vi "ke37xx DAC-Totalizer Calibration.vi"() -> ()   [LabVIEW 2009, in "Keithley 3700 Series.lvlib"]
doc: "This VI provides a way to calibrate the 3750 Digital I/O Card's DAC and totalizer channels. Ensure all inputs to the channels being calibrated are disconnected."
uses:
  <instrlib>/Keithley 3706/Keithley 3700 Series.lvlib
panel:
  out "Calibration Failed":bool=TRUE
  out "Calibration Completed":bool
  out "error out":errorcluster
  in  "Calibration Password":string
  in  "Channel Type":enum32{"Radio Selection 1", "Radio Selection 2"}(radio)
  in  "Channel to Calibrate":string
  in  "VISA Resource Name":refnum<visa-resource-name>
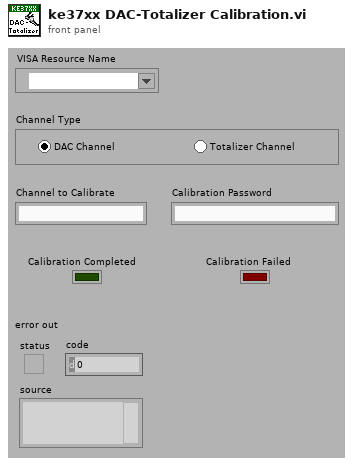
[diagram p1: front panel]
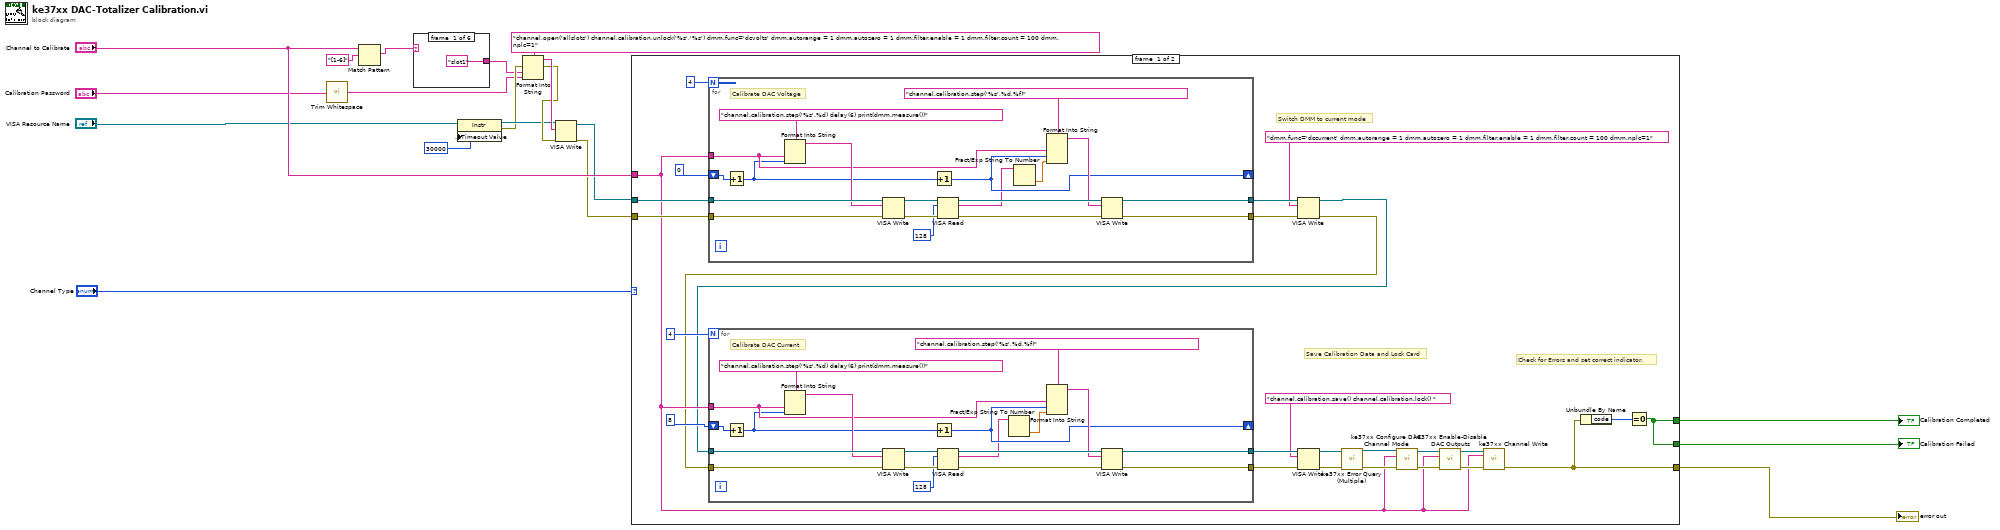
[diagram p0: block diagram]
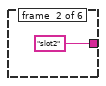
[diagram p2: hidden frame]
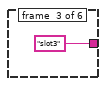
[diagram p3: hidden frame]
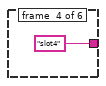
[diagram p4: hidden frame]
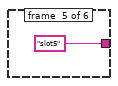
[diagram p5: hidden frame]
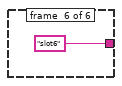
[diagram p6: hidden frame]
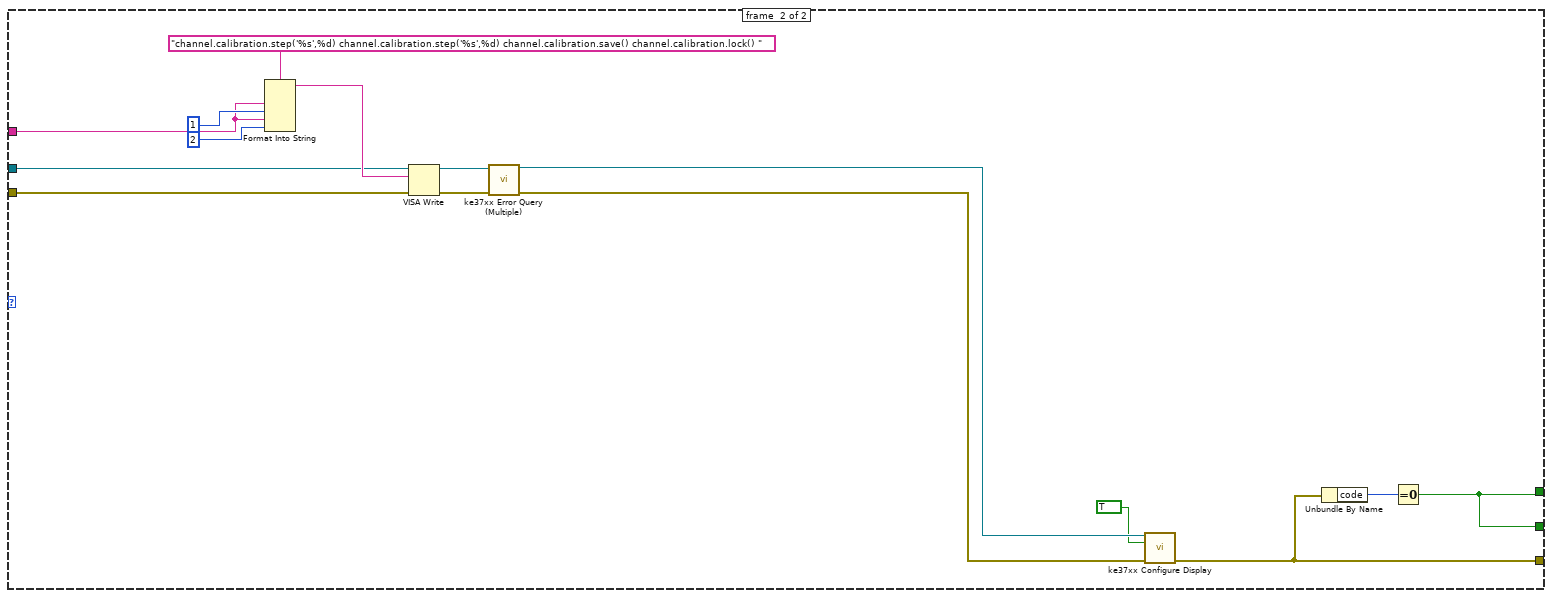
[diagram p7: hidden frame]
diagram:
  n1 = call <vilib>:"Trim Whitespace.vi"("string"="Calibration Password") -> ("trimmed string"=w1:string)  [unwired: 1 in]
  n2 = Match Pattern(string="Channel to Calibrate", regular expression="[1-6]") -> (match substring=w6:string)  [unwired: 4 out]
  n3 = case shown="\"4\"" w6 {
    tunnel: ["slot1" "slot2" "slot3" "slot4" "slot5" "slot6"] -> w5
    frame #0 {
    }
    frame #1 {
    }
    frame #2 {
    }
    frame #3 {
    }
    frame #4 {
    }
    frame #5 {
    }
  }
  n4 = property class="Instr"(reference="VISA Resource Name", "General Settings:Timeout Value"=u32 30000) -> (reference out=w9:refnum<visa-resource-name>, error out=w8:errorcluster)  [unwired: 1 in]
  n5 = Format Into String(format string="channel.open('allslots') channel.calibration.unlock('%s','%s') dmm.func='dcvolts' dmm.autorange = 1 dmm.autozero = 1 dmm.filter.enable = 1 dmm.filter.count = 100 dmm.nplc=1", error in=w8, w5, w1) -> (resulting string=w13:string, error out=w10:errorcluster)  [unwired: 1 in]
  n6 = VISA Write(VISA resource name=w9, write buffer=w13, error in (no error)=w10) -> (VISA resource name out=w4:refnum<visa-resource-name>, error out=w3:errorcluster)  [unwired: 1 out]
  n7 = case shown="\"Radio Selection 1\", Default" "Channel Type" {
    tunnel: w3 -> [w50 w101]
    tunnel: w4 -> [w49 w102]
    tunnel: "Channel to Calibrate" -> [w32 w96]
    tunnel: [w26 w93] -> w14
    tunnel: [w27 w94] -> w16
    tunnel: [w27 w94] -> w15
    frame #0 {
      # "Check for Errors and set correct indicator."
      # "Switch DMM to current mode"
      # "Save Calibration Data and Lock Card"
      n8 = for {
        N: 4 -> [_]
        tunnel: [w71] -> w46
        tunnel: w50 -> [w89]
        tunnel: w49 -> [w88]
        tunnel: w32 -> [w78]
        shift-right: [w77] -> _
        shift-left: 0 -> [w75]
        tunnel: [w72] -> w47
        # "Calibrate DAC Voltage"
        n9 = Increment(x=w75) -> (x+1=w76:i32)
        n10 = Format Into String(format string="channel.calibration.step('%s',%d) delay(6) print(dmm.measure())", w78, w76) -> (resulting string=w86:string)  [unwired: 2 in, 1 out]
        n11 = VISA Write(VISA resource name=w88, write buffer=w86, error in (no error)=w89) -> (VISA resource name out=w85:refnum<visa-resource-name>, error out=w84:errorcluster)  [unwired: 1 out]
        n12 = Increment(x=w76) -> (x+1=w77:i32)
        n13 = VISA Read(VISA resource name=w85, byte count=128, error in (no error)=w84) -> (VISA resource name out=w82:refnum<visa-resource-name>, read buffer=w74:string, error out=w81:errorcluster)  [unwired: 1 out]
        n14 = Fract/Exp String To Number(string=w74) -> (number=w73:dbl)  [unwired: 4 out]
        n15 = Format Into String(format string="channel.calibration.step('%s',%d,%f)", w78, w77, w73) -> (resulting string=w79:string)  [unwired: 2 in, 1 out]
        n16 = VISA Write(VISA resource name=w82, write buffer=w79, error in (no error)=w81) -> (VISA resource name out=w72:refnum<visa-resource-name>, error out=w71:errorcluster)  [unwired: 1 out]
      }
      n17 = VISA Write(VISA resource name=w47, write buffer="dmm.func='dccurrent' dmm.autorange = 1 dmm.autozero = 1 dmm.filter.enable = 1 dmm.filter.count = 100 dmm.nplc=1", error in (no error)=w46) -> (VISA resource name out=w29:refnum<visa-resource-name>, error out=w28:errorcluster)  [unwired: 1 out]
      n18 = for {
        N: 4 -> [_]
        tunnel: [w53] -> w31
        tunnel: w28 -> [w70]
        tunnel: w29 -> [w69]
        tunnel: w32 -> [w59]
        shift-right: [w58] -> _
        shift-left: 8 -> [w56]
        tunnel: [w54] -> w40
        # "Calibrate DAC Current"
        n19 = Increment(x=w56) -> (x+1=w57:i32)
        n20 = Format Into String(format string="channel.calibration.step('%s',%d) delay(6) print(dmm.measure())", w59, w57) -> (resulting string=w67:string)  [unwired: 2 in, 1 out]
        n21 = VISA Write(VISA resource name=w69, write buffer=w67, error in (no error)=w70) -> (VISA resource name out=w66:refnum<visa-resource-name>, error out=w65:errorcluster)  [unwired: 1 out]
        n22 = Increment(x=w57) -> (x+1=w58:i32)
        n23 = VISA Read(VISA resource name=w66, byte count=128, error in (no error)=w65) -> (VISA resource name out=w63:refnum<visa-resource-name>, read buffer=w55:string, error out=w62:errorcluster)  [unwired: 1 out]
        n24 = Fract/Exp String To Number(string=w55) -> (number=w52:dbl)  [unwired: 4 out]
        n25 = Format Into String(format string="channel.calibration.step('%s',%d,%f)", w59, w58, w52) -> (resulting string=w60:string)  [unwired: 2 in, 1 out]
        n26 = VISA Write(VISA resource name=w63, write buffer=w60, error in (no error)=w62) -> (VISA resource name out=w54:refnum<visa-resource-name>, error out=w53:errorcluster)  [unwired: 1 out]
      }
      n27 = VISA Write(VISA resource name=w40, write buffer="channel.calibration.save() channel.calibration.lock() ", error in (no error)=w31) -> (VISA resource name out=w41:refnum<visa-resource-name>, error out=w42:errorcluster)  [unwired: 1 out]
      n28 = call <instrlib>:"ke37xx Error Query (Multiple).vi"("VISA resource name"=w41, "error in (no error)"=w42) -> ("VISA resource name out"=w38:refnum<visa-resource-name>, "error out"=w37:errorcluster)  [unwired: 12 out]
      n29 = call <instrlib>:"ke37xx Configure DAC Channel Mode.vi"("error in (no error)"=w37, "DAC Channels"=w32, "VISA Resource Name"=w38) -> ("error out"=w35:errorcluster, "VISA Resource Name Out"=w36:refnum<visa-resource-name>)  [unwired: 1 in, 6 out]
      n30 = call <instrlib>:"ke37xx Enable-Disable DAC Outputs.vi"("error in (no error)"=w35, "Channel"=w32, "VISA Resource Name"=w36) -> ("error out"=w33:errorcluster, "VISA Resource Name Out"=w34:refnum<visa-resource-name>)  [unwired: 1 in, 6 out]
      n31 = call <instrlib>:"ke37xx Channel Write.vi"("VISA Resource Name"=w34, "Channel"=w32, "error in (no error)"=w33) -> ("error out"=w26:errorcluster)  [unwired: 2 in, 10 out]
      n32 = Unbundle By Name(w26) -> ("code"=w30:i32)
      n33 = Equal To 0?(x=w30) -> (x = 0?=w27:bool)
    }
    frame #1 {
      n34 = Format Into String(format string="channel.calibration.step('%s',%d) channel.calibration.step('%s',%d) channel.calibration.save() channel.calibration.lock() ", w96, 1, w96, 2) -> (resulting string=w103:string)  [unwired: 2 in, 1 out]
      n35 = VISA Write(VISA resource name=w102, write buffer=w103, error in (no error)=w101) -> (VISA resource name out=w99:refnum<visa-resource-name>, error out=w98:errorcluster)  [unwired: 1 out]
      n36 = call <instrlib>:"ke37xx Error Query (Multiple).vi"("VISA resource name"=w99, "error in (no error)"=w98) -> ("VISA resource name out"=w91:refnum<visa-resource-name>, "error out"=w92:errorcluster)  [unwired: 12 out]
      n37 = call <instrlib>:"ke37xx Configure Display.vi"("VISA Resource Name"=w91, "Clear Display (False)"=TRUE, "error in (no error)"=w92) -> ("error out"=w93:errorcluster)  [unwired: 11 in, 1 out]
      n38 = Unbundle By Name(w93) -> ("code"=w95:i32)
      n39 = Equal To 0?(x=w95) -> (x = 0?=w94:bool)
    }
  }
  "error out" <- w14
  "Calibration Completed" <- w16
  "Calibration Failed" <- w15
